vi "L12_1.0.vi"   [LabVIEW 2012]
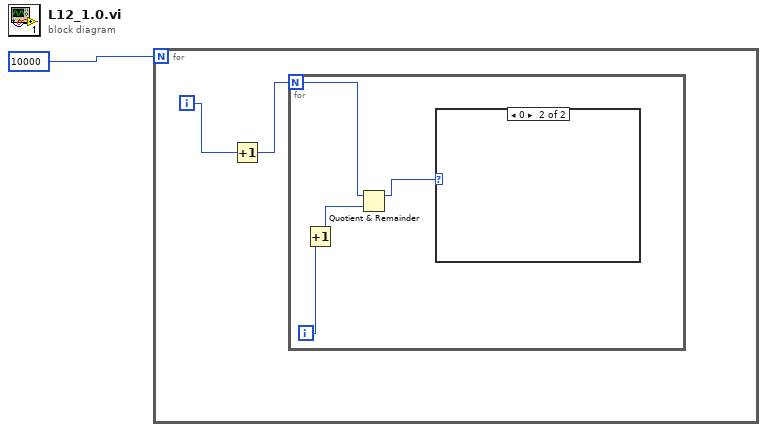
[diagram p0: block diagram]
diagram:
  n1 = for {
    N: 10000 -> [_]
    i -> [w3]
    n2 = Increment(x=w3) -> (x+1=w2:i32)
    n3 = for {
      N: w2 -> [w7]
      i -> [w6]
      n4 = Increment(x=w6) -> (x+1=w5:i32)
      n5 = Quotient & Remainder(x=w7, y=w5) -> (x-y*floor(x/y)=w4:i32)  [unwired: 1 out]
      n6 = case shown="0" w4 {
        frame Default {
        }
        frame 0 {
        }
      }
    }
  }
